vi "G#Interface_Create.vi"(0 "reference in":refnum<class "G#Interface.lvclass">, 2 "G#Object in":refnum<class "G#Object.lvclass">, 5 "error in (no error)":errorcluster) -> (14 "reference out":refnum<class "G#Interface.lvclass">, 19 "error out":errorcluster)   [LabVIEW 2020, in "G#Interface.lvclass"]
doc: "Creates the G#Interface for the G#Object."
uses:
  G#Interface.lvclass
  G#Object/G#Object.lvclass
  G#Interface.lvclass/G#Interface.ctl
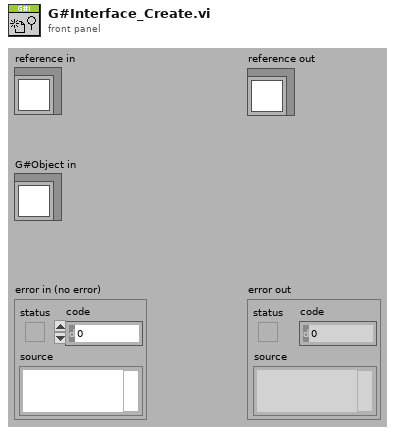
[diagram p1: front panel]
types:
  T1 = typedef "G#Object.lvclass/G#Object_ClassHierarchy.ctl" = cluster{"ClassName":string, "FullClassName":string, "ClassPath":path, "IsLeaf":bool}
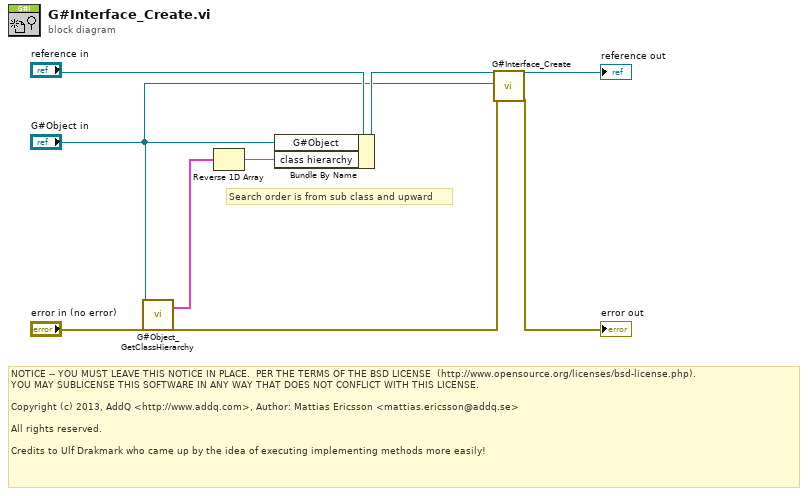
[diagram p0: block diagram]
diagram:
  # "NOTICE -- YOU MUST LEAVE THIS NOTICE IN PLACE.  PER THE TERMS OF THE BSD LICENSE  (http://www.opensource.org/licenses/bsd-license.php).\nYOU MAY SUBLICENSE THIS SOFTWARE IN ANY WAY THAT DOES NOT CONFLICT WITH THIS LICENSE.\n\nCopyright (c) 2013, AddQ <http://www.addq.com>, Author: Mattias Ericsson <mattias.ericsson@addq.se>\n\nAll rights reserved.\n\nCredits to Ulf Drakmark who came up by the idea of executing implementing methods more easily!"
  # "Search order is from sub class and upward"
  n1 = call "G#Object_GetClassHierarchy.vi"("reference in"="G#Object in", "error in (no error)"="error in (no error)") -> ("class hierarchy"=w7:T1[], "error out"=w5:errorcluster)  [unwired: 15 in, 1 out]
  n2 = Reverse 1D Array(array=w7) -> (reversed array=w6:T1[])
  n3 = Bundle By Name(cluster="reference in", "G#Object"="G#Object in", "class hierarchy"=w6) -> (w3:refnum<class "G#Interface.lvclass">)
  n4 = call-parent "G#Interface_Create.vi"("reference in"=w3, "G#Object in"="G#Object in", "error in (no error)"=w5) -> ("reference out"=→"reference out":refnum<class "G#Interface.lvclass">, "error out"=→"error out":errorcluster)  [unwired: 15 in]
